vi "Camera Initialization.vi"(11 "Camera Number":i32) -> (0 "error out":errorcluster, 3 "Cluster":cluster{"Session Out":T1, "Camera Number":i32})   [LabVIEW 2016]
uses:
  <vilib>/userdefined/High Color/IMAQdx.ctl
  <vilib>/vision/driver/NI_Vision_Acquisition_Software.lvlib
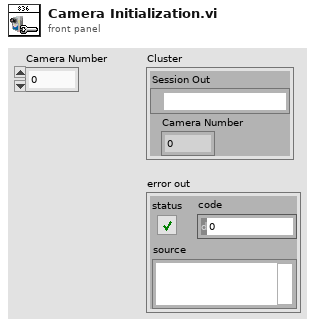
[diagram p1: front panel]
types:
  T1 = typedef "IMAQdx.ctl" = refnum<k21>
  T2 = cluster{"Type":u32, "Version":u32, "Flags":u32, "SerialNumberHigh":u32, "SerialNumberLow":u32, "BusType":u32, "InterfaceName":string, "VendorName":string, "ModelName":string, "CameraFileName":string, "CameraAttributeURL":string}[]
  T3 = cluster{"Type":u32, "Version":u32, "Flags":u32, "SerialNumberHigh":u32, "SerialNumberLow":u32, "BusType":u32, "InterfaceName":string, "VendorName":string, "ModelName":string, "CameraFileName":string, "CameraAttributeURL":string}
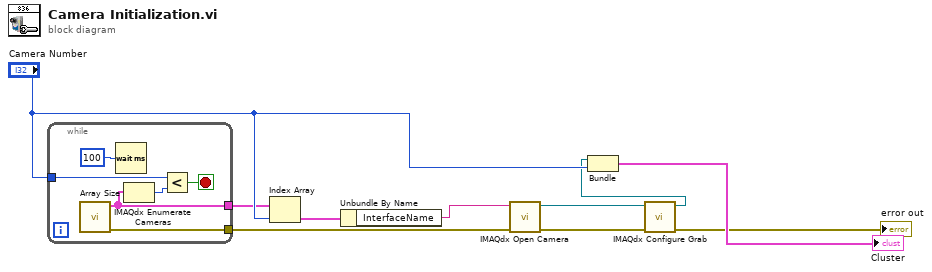
[diagram p0: block diagram]
diagram:
  n1 = while {
    tunnel: [w15] -> w1
    tunnel: [w16] -> w5
    tunnel: "Camera Number" -> [w13]
    stop <- w12 stop-if-true
    n2 = call <vilib>:"IMAQdx Enumerate Cameras.vi"() -> ("error out"=w16:errorcluster, "Camera Information Array"=w15:T2)  [unwired: 10 in]
    n3 = Wait (ms)(milliseconds to wait=u32 100) -> ()  [unwired: 1 out]
    n4 = Array Size(array=w15) -> (size(s)=w14:i32)
    n5 = Less?(x=w13, y=w14) -> (x < y?=w12:bool)
  }
  n6 = Index Array(array=w1, index="Camera Number") -> (element=w2:T3)
  n7 = Unbundle By Name(w2) -> ("InterfaceName"=w3:string)
  n8 = call <vilib>:"IMAQdx Open Camera.vi"("error in"=w5, "Session In"=w3) -> ("error out"=w6:errorcluster, "Session Out"=w4:T1)  [unwired: 8 in]
  n9 = call <vilib>:"IMAQdx Configure Grab.vi"("error in"=w6, "Session In"=w4) -> ("error out"=→"error out":errorcluster, "Session Out"=w8:T1)  [unwired: 8 in]
  n10 = Bundle("Session Out"=w8, "Camera Number"="Camera Number") -> (→"Cluster":cluster{"Session Out":T1, "Camera Number":i32})  [unwired: 1 in]
